vi "Root Parallel Operation.vi"(8 "error in (no error)":errorcluster, 9 "Stop Notifier In":refnum<notifier>, 11 "Parallel Operation Root Actor in":refnum<class "Parallel Operation Root Actor.lvclass">) -> (0 "error out":errorcluster, 1 "Stop Notifier Out":refnum<notifier>, 3 "Parallel Operation Root Actor out":refnum<class "Parallel Operation Root Actor.lvclass">, 4 "Notifier Status":bool)   [LabVIEW 2024, in "Parallel Operation Root Actor.lvclass"]
uses:
  Parallel Operation Root Actor.lvclass
  Parallel Operation Root Actor.lvclass/Parallel Operation Root Actor.ctl
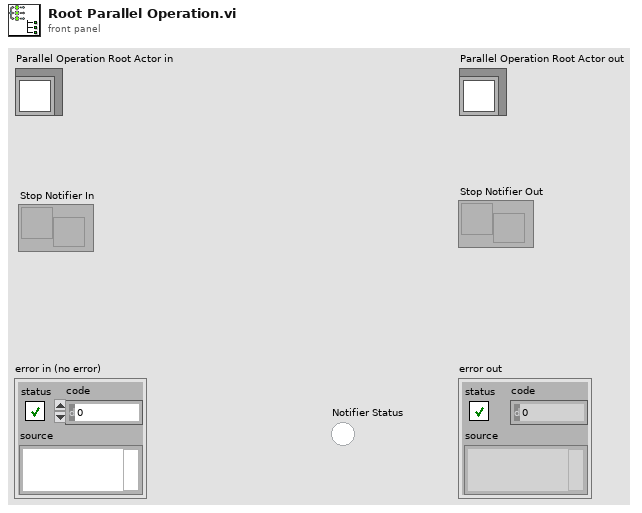
[diagram p1: front panel]
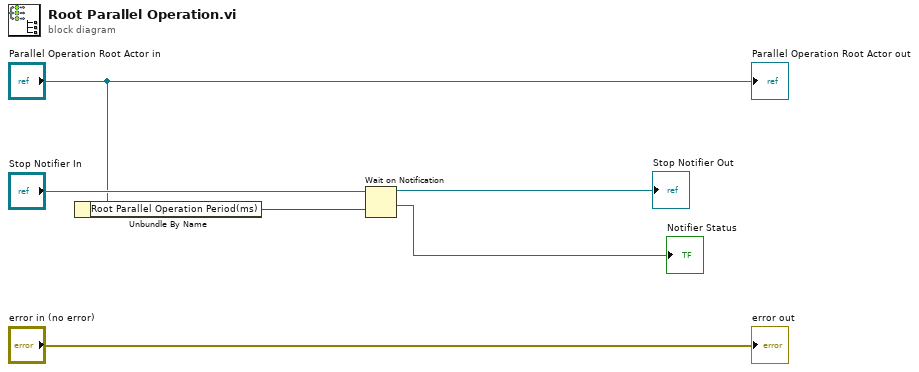
[diagram p0: block diagram]
diagram:
  n1 = Unbundle By Name("Parallel Operation Root Actor in") -> ("Root Parallel Operation Period(ms)"=w1:i32)
  n2 = Wait on Notification(notifier="Stop Notifier In", timeout in ms (-1)=w1) -> (notifier out=→"Stop Notifier Out":refnum<notifier>, timed out?=→"Notifier Status":bool)  [unwired: 2 in, 2 out]
  "error out" <- "error in (no error)"
  "Parallel Operation Root Actor out" <- "Parallel Operation Root Actor in"
